vi "Initialize Rigol.vi"(6 "error in":errorcluster caption="error in (no error)", 9 "MAX name":string) -> (0 "error out":errorcluster, 3 "VISA resource name out":refnum<visa-resource-name>)   [LabVIEW 2023]
uses:
  <instrlib>/RIGOL DP800 Series/RIGOL DP800 Series.lvlib
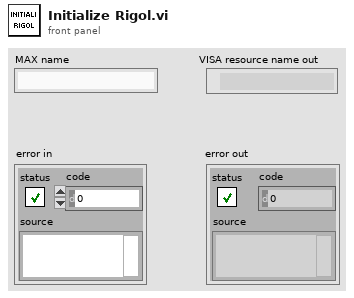
[diagram p1: front panel]
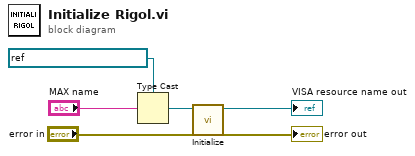
[diagram p0: block diagram]
diagram:
  n1 = Type Cast(type=refnum<visa-resource-name> "Rigol_DP800_CHMB1" ("VISA resource name"), x="MAX name") -> (*(type *) &x=w3:refnum<visa-resource-name>)
  n2 = call <instrlib>:"Initialize.vi"("error in (no error)"="error in", "VISA resource name"=w3) -> ("error out"=→"error out":errorcluster, "VISA resource name out"=→"VISA resource name out":refnum<visa-resource-name>)  [unwired: 8 in]
